vi "Set Label Position.vi"(6 "Variant in":variant, 7 "Shift Pressed?":bool, 8 "error in (no error)":errorcluster, 10 "QD Combo Box Ref":refnum<vi>, 11 "QD Launch VI Ref":refnum<vi>) -> (0 "error out":errorcluster, 4 "Variant out":variant)   [LabVIEW 2015]
doc: "Default Shortcut - [2]"
uses:
  <vilib>/Utility/config.llb/Read Key (String).vi
  <vilib>/Utility/config.llb/NI_LVConfig.lvlib
panel:
  in  "Undo Name":string="Quick Drop Keyboard Shortcut"
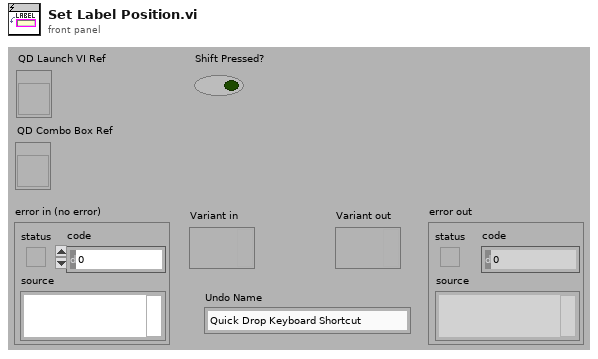
[diagram p1: front panel]
types:
  T1 = typedef "NI_LVConfig.lvlib/Config Data RefNum.ctl" = refnum<k1>
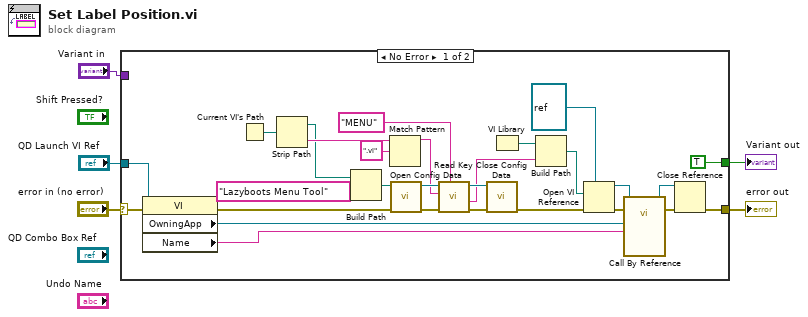
[diagram p0: block diagram]
diagram:
  n1 = case shown="No Error" "error in (no error)" {
    selector: "error in (no error)" -> [w33 w34]
    tunnel: [w32 w34] -> w4
    tunnel: "QD Launch VI Ref" -> [w31 _]
    tunnel: [TRUE _] -> w2
    tunnel: "Variant in" -> [_ _]
    frame No Error {
      n2 = property class="VI"(reference=w31, error in=w33) -> (error out=w11:errorcluster, "OwningApp"=w13:refnum<vi>, "Name"=w12:string)  [unwired: 1 out]
      n3 = Current VI's Path() -> (path=w27:path)
      n4 = Strip Path(path=w27) -> (stripped path=w9:path, name=w19:string)
      n5 = Build Path(base path=w9, name or relative path="Lazyboots Menu Tool") -> (appended path=w25:path)
      n6 = Match Pattern(string=w19, regular expression=".vi") -> (before substring=w18:string)  [unwired: 4 out]
      n7 = call <vilib>:"Open Config Data.vi"("error in (no error)"=w11, "configuration file path"=w25) -> ("error out"=w23:errorcluster, "refnum"=w24:T1)  [unwired: 7 in, 1 out]
      n8 = call-poly <vilib>:"Read Key.vi"("section"="MENU", "error in (no error)"=w23, "key"=w18, "refnum"=w24) -> ("error out"=w20:errorcluster, "value"=w15:string, "refnum out"=w21:T1)  [unwired: 2 in, 3 out]
      n9 = call <vilib>:"Close Config Data.vi"("error in (no error)"=w20, "refnum"=w21) -> ("error out"=w10:errorcluster)  [unwired: 1 in, 8 out]
      n10 = VI Library() -> (path=w14:path)
      n11 = Build Path(base path=w14, name or relative path=w15) -> (appended path=w16:path)
      n12 = Open VI Reference(type specifier VI Refnum (for type only)=refnum<vi> refnum, vi path=w16, error in (no error)=w10) -> (vi reference=w7:refnum<vi>, error out=w29:errorcluster)  [unwired: 3 out]
      n13 = call-by-ref "?"(reference=w7, error in=w29, "VI Path"=w12, "Application Reference"=w13) -> (reference out=w8:refnum<vi>, error out=w28:errorcluster)  [unwired: 9 in, 1 out]
      n14 = Close Reference(reference=w8, error in (no error)=w28) -> (error out=w32:errorcluster)
    }
    frame Error {
    }
  }
  "error out" <- w4
  "Variant out" <- w2
